vi "二分法-日期时间插入位置输出.vi"(8 "单个-日期时间组合":i32[](array[numeric]), 11 "数组-日期时间组合":i32[][](array[numeric])) -> (0 "插入此索引处":i32)   [LabVIEW 2013]
panel:
  out "最近索引":i32
  out "s? t:f":enum16{"从小到大", "从大到小"}(ring)
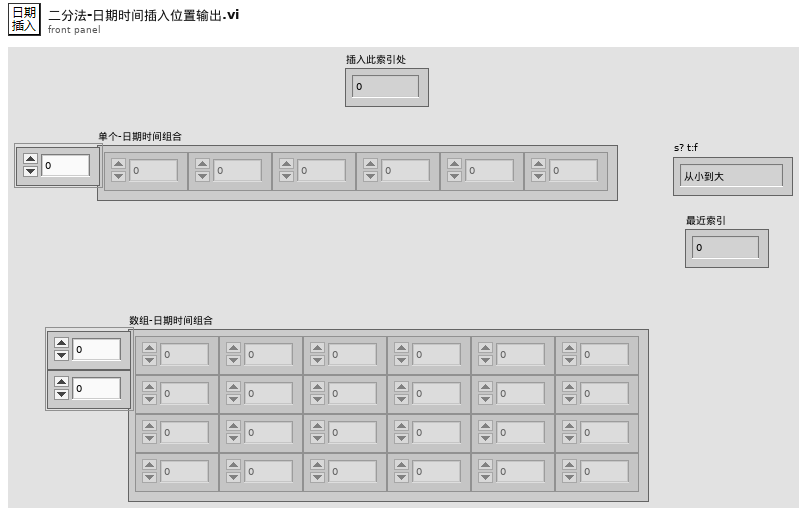
[diagram p1: front panel]
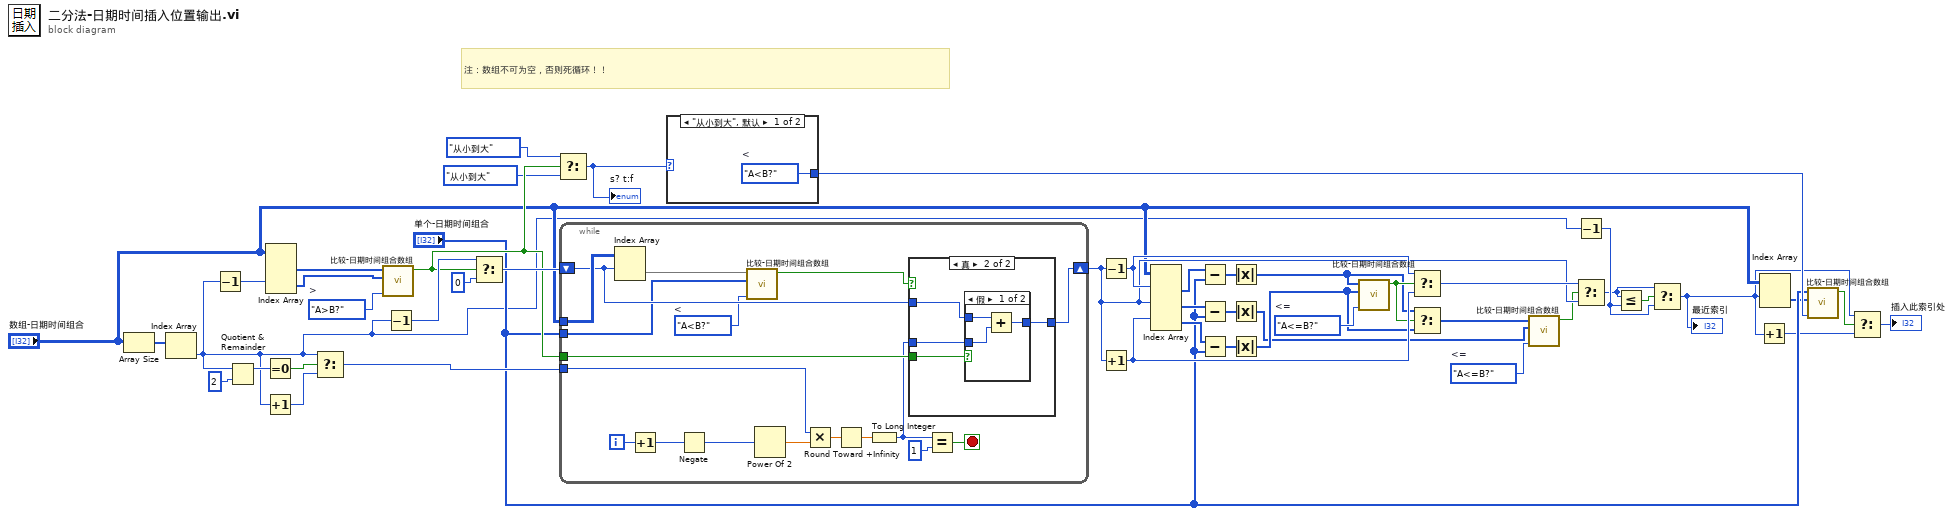
[diagram p0: block diagram]
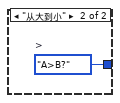
[diagram p2: hidden frame]
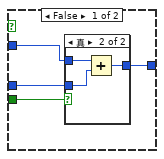
[diagram p3: hidden frame]
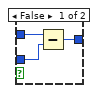
[diagram p4: hidden frame]
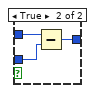
[diagram p5: hidden frame]
diagram:
  w16 = enum16{"A>B?", "A<B?", "A>=B?", "A<=B?", "A=B?"}."A<=B?"  # <=
  w20 = enum16{"A>B?", "A<B?", "A>=B?", "A<=B?", "A=B?"}."A<=B?"  # <=
  w24 = enum16{"A>B?", "A<B?", "A>=B?", "A<=B?", "A=B?"}."A>B?"  # >
  # "注：数组不可为空，否则死循环！！"
  n1 = Array Size(array="数组-日期时间组合") -> (size(s)=w25:i32[])
  n2 = Index Array(array=w25) -> (element=w1:i32)  [unwired: 1 in]
  n3 = Decrement(x=w1) -> (x-1=w47:i32)
  n4 = Quotient & Remainder(x=w1, y=2) -> (x-y*floor(x/y)=w45:i32)  [unwired: 1 out]
  n5 = Equal To 0?(x=w45) -> (x = 0?=w44:bool)
  n6 = Increment(x=w1) -> (x+1=w43:i32)
  n7 = Index Array(array="数组-日期时间组合", index (row) #2=w47) -> (element #1=w22:i32[], element #2=w21:i32[])  [unwired: 3 in]
  n8 = Select(t=w1, s=w44, f=w43) -> (s? t:f=w42:i32)
  n9 = call "比较-日期时间组合数组.vi"("比较模式"=w24, "日期时间B"=w21, "日期时间A"=w22) -> ("结果"=w23:bool)  [unwired: 8 in]
  n10 = Decrement(x=w1) -> (x-1=w28:i32)
  n11 = Select(t=w28, s=w23, f=0 ("索引")) -> (s? t:f=w26:i32)
  n12 = Select(t=enum16{"从小到大", "从大到小"}."从小到大" ("s? t:f"), s=w23, f=enum16{"从小到大", "从大到小"}."从小到大" ("s? t:f")) -> (s? t:f=w9:enum16{"从小到大", "从大到小"})
  "s? t:f" <- w9
  n13 = while {
    tunnel: "数组-日期时间组合" -> [w65]
    tunnel: "单个-日期时间组合" -> [w49]
    shift-right: [w61] -> w30
    shift-left: w26 -> [w62]
    tunnel: w42 -> [w54]
    tunnel: w23 -> [w64]
    i -> [w57]
    stop <- w58 stop-if-true
    w50 = enum16{"A>B?", "A<B?", "A>=B?", "A<=B?", "A=B?"}."A<B?"  # <
    n14 = Index Array(array=w65, index (row)=w62) -> (element=w48:i32[])  [unwired: 1 in]
    n15 = Increment(x=w57) -> (x+1=w56:i32)
    n16 = Negate(x=w56) -> (-x=w55:i32)
    n17 = call "比较-日期时间组合数组.vi"("比较模式"=w50, "日期时间B"=w49, "日期时间A"=w48) -> ("结果"=w51:bool)  [unwired: 8 in]
    n18 = Power Of 2(x=w55) -> (2^x=w53:dbl)
    n19 = Multiply(x=w54, y=w53) -> (x*y=w52:dbl)
    n20 = Round Toward +Infinity(x=w52) -> (ceil(x): smallest int >= x=w63:dbl)
    n21 = To Long Integer(number=w63) -> (32bit integer=w60:i32)
    n22 = case shown="真" w51 {
      tunnel: w64 -> [w69 w79]
      tunnel: w60 -> [w68 w78]
      tunnel: w62 -> [w67 w77]
      tunnel: [w66 w76] -> w61
      frame False {
        n23 = case shown="真" w69 {
          tunnel: w68 -> [w72 w75]
          tunnel: w67 -> [w71 w74]
          tunnel: [w70 w73] -> w66
          frame False {
            n24 = Subtract(x=w71, y=w72) -> (x-y=w70:i32)
          }
          frame True {
            n25 = Add(x=w74, y=w75) -> (x+y=w73:i32)
          }
        }
      }
      frame True {
        n26 = case shown="假" w79 {
          tunnel: w78 -> [w82 w85]
          tunnel: w77 -> [w81 w84]
          tunnel: [w80 w83] -> w76
          frame False {
            n27 = Add(x=w81, y=w82) -> (x+y=w80:i32)
          }
          frame True {
            n28 = Subtract(x=w84, y=w85) -> (x-y=w83:i32)
          }
        }
      }
    }
    n29 = Equal?(x=w60, y=1) -> (x = y?=w58:bool)
  }
  n30 = case shown="\"从小到大\", 默认" w9 {
    tunnel: [w86 w87] -> w8
    frame "从小到大", Default {
      w86 = enum16{"A>B?", "A<B?", "A>=B?", "A<=B?", "A=B?"}."A<B?"  # <
    }
    frame "从大到小" {
      w87 = enum16{"A>B?", "A<B?", "A>=B?", "A<=B?", "A=B?"}."A>B?"  # >
    }
  }
  n31 = Decrement(x=w30) -> (x-1=w33:i32)
  n32 = Increment(x=w30) -> (x+1=w32:i32)
  n33 = Index Array(array="数组-日期时间组合", index (row) #1=w33, index (row) #2=w30, index (row) #3=w32) -> (element #1=w41:i32[], element #2=w34:i32[], element #3=w36:i32[])  [unwired: 3 in]
  n34 = Subtract(x=w41, y="单个-日期时间组合") -> (x-y=w39:i32[])
  n35 = Subtract(x=w34, y="单个-日期时间组合") -> (x-y=w35:i32[])
  n36 = Subtract(x=w36, y="单个-日期时间组合") -> (x-y=w40:i32[])
  n37 = Absolute Value(x=w39) -> (abs(x)=w18:i32[])
  n38 = Absolute Value(x=w35) -> (abs(x)=w13:i32[])
  n39 = Absolute Value(x=w40) -> (abs(x)=w17:i32[])
  n40 = call "比较-日期时间组合数组.vi"("比较模式"=w20, "日期时间B"=w17, "日期时间A"=w18) -> ("结果"=w19:bool)  [unwired: 8 in]
  n41 = Select(t=w33, s=w19, f=w32) -> (s? t:f=w31:i32)
  n42 = Select(t=w18, s=w19, f=w17) -> (s? t:f=w14:i32[])
  n43 = call "比较-日期时间组合数组.vi"("比较模式"=w16, "日期时间B"=w13, "日期时间A"=w14) -> ("结果"=w15:bool)  [unwired: 8 in]
  n44 = Decrement(x=w1) -> (x-1=w37:i32)
  n45 = Select(t=w31, s=w15, f=w30) -> (s? t:f=w29:i32)
  n46 = Less Or Equal?(x=w29, y=w37) -> (x <= y?=w38:bool)
  n47 = Select(t=w29, s=w38, f=w37) -> (s? t:f=w4:i32)
  "最近索引" <- w4
  n48 = Increment(x=w4) -> (x+1=w3:i32)
  n49 = Index Array(array="数组-日期时间组合", index (row)=w4) -> (element=w6:i32[])  [unwired: 1 in]
  n50 = call "比较-日期时间组合数组.vi"("比较模式"=w8, "日期时间B"=w6, "日期时间A"="单个-日期时间组合") -> ("结果"=w5:bool)  [unwired: 8 in]
  n51 = Select(t=w4, s=w5, f=w3) -> (s? t:f=→"插入此索引处":i32)
